vi "test compare match pattern.vi"() -> (3 "pass?":bool)   [LabVIEW 2019, in "ANODE Tests.lvlib"]
uses:
  ANODE Tests.lvlib
panel:
  out "not match invalid pattern?":bool
  out "mismatch?":bool
  out "not match?":bool
  out "match?":bool
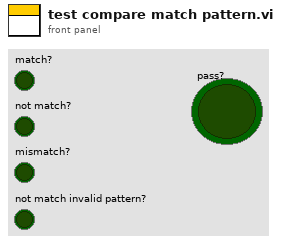
[diagram p1: front panel]
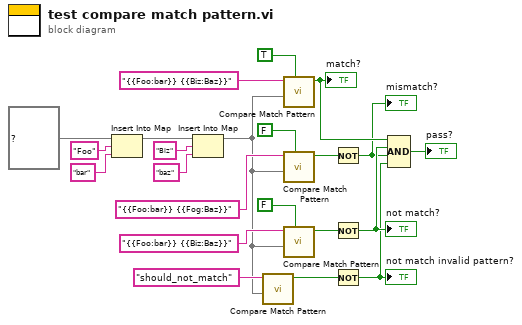
[diagram p0: block diagram]
diagram:
  n1 = Insert Into Map(map in=map{string, string} {} ("substitutions"), key="Foo", value="bar" ("key")) -> (map out=w18:map{string, string})  [unwired: 2 out]
  n2 = Insert Into Map(map in=w18, key="Biz", value="baz" ("key")) -> (map out=w1:map{string, string})  [unwired: 2 out]
  n3 = call "Compare Match Pattern.vi"("substitutions"=w1, "string to match"="should_not_match") -> ("match?"=w4:bool)  [unwired: 8 in, 1 out]
  n4 = call "Compare Match Pattern.vi"("ignore case? (F)"=TRUE, "substitutions"=w1, "string to match"="{{Foo:bar}} {{Biz:Baz}}") -> ("match?"=w8:bool)  [unwired: 7 in, 1 out]
  "match?" <- w8
  n5 = call "Compare Match Pattern.vi"("ignore case? (F)"=FALSE, "substitutions"=w1, "string to match"="{{Foo:bar}} {{Fog:Baz}}") -> ("match?"=w9:bool)  [unwired: 7 in, 1 out]
  n6 = call "Compare Match Pattern.vi"("ignore case? (F)"=FALSE, "substitutions"=w1, "string to match"="{{Foo:bar}} {{Biz:Baz}}") -> ("match?"=w12:bool)  [unwired: 7 in, 1 out]
  n7 = Not(x=w9) -> (.not. x?=w6:bool)
  "mismatch?" <- w6
  n8 = Not(x=w12) -> (.not. x?=w7:bool)
  "not match?" <- w7
  n9 = Not(x=w4) -> (.not. x?=w3:bool)
  "not match invalid pattern?" <- w3
  n10 = Compound Arithmetic op=AND(w8, w7, w6, w3) -> (→"pass?":bool)
